vi "Authenticate.vi"(8 "error in (no error)":errorcluster, 10 "Authentication Inputs":T2, 11 "SOL Auth in":refnum<class "SOL Auth.lvclass">) -> (0 "error out":errorcluster, 2 "Authentication Outputs":T1, 3 "SOL Auth out":refnum<class "SOL Auth.lvclass">)   [LabVIEW 2020, in "Summer of LabVIEW.lvlib" / "SOL Auth.lvclass"]
uses:
  SOL Auth.lvclass
  <vilib>/IlluminatedG/IG HTTP Server/HTTP Server/Authentication Inputs.ctl
  <vilib>/IlluminatedG/IG HTTP Server/HTTP Server/Session/Session.lvclass
  <vilib>/IlluminatedG/IG HTTP Utils/HTTP Utils/Request/Request.lvclass
  <vilib>/IlluminatedG/IG HTTP Server/HTTP Server/User Provider/User Provider.lvclass
  <vilib>/IlluminatedG/IG HTTP Server/HTTP Server/Password Encoder/Password Encoder.lvclass
  <vilib>/IlluminatedG/IG HTTP Server/HTTP Server/Authentication Outputs.ctl
  <vilib>/IlluminatedG/IG HTTP Server/HTTP Server/User/User.lvclass
  Data Types/Login JSON.ctl
  Summer of LabVIEW.lvlib
  <vilib>/IlluminatedG/IG HTTP Server/HTTP Server/HTTP Server.lvlib
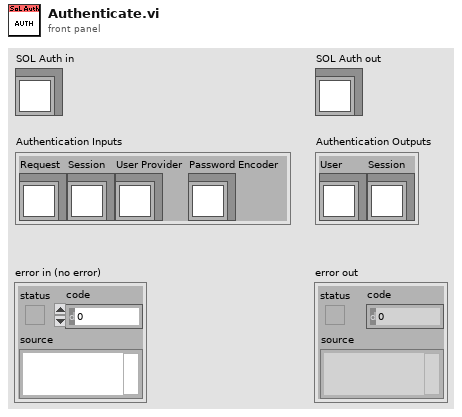
[diagram p1: front panel]
types:
  T1 = typedef "HTTP Server.lvlib/Authentication Outputs.ctl" = cluster{"User":refnum<class "User.lvclass">, "Session":refnum<class "Session.lvclass">}
  T2 = typedef "HTTP Server.lvlib/Authentication Inputs.ctl" = cluster{"Request":refnum<class "Request.lvclass">, "Session":refnum<class "Session.lvclass">, "User Provider":refnum<class "User Provider.lvclass">, "Password Encoder":refnum<class "Password Encoder.lvclass">}
  T3 = typedef "Summer of LabVIEW.lvlib/Login JSON.ctl" = cluster{"Email":string, "Password":string, "CSRF":string}
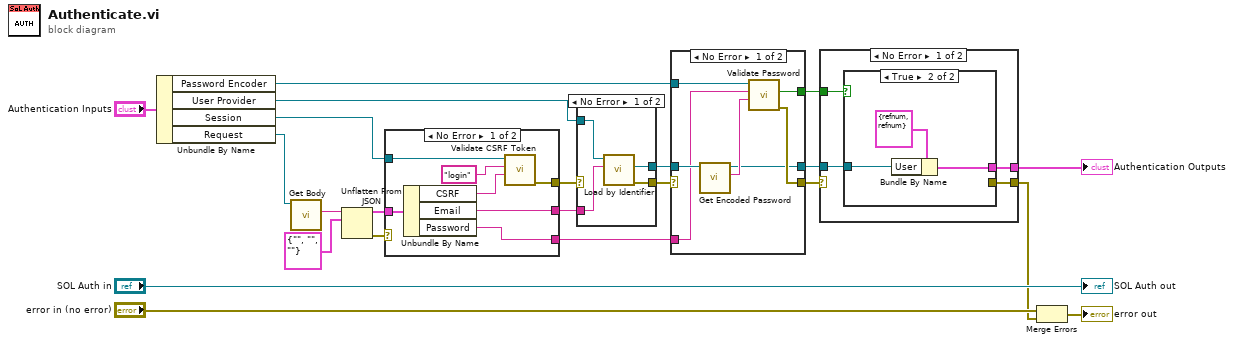
[diagram p0: block diagram]
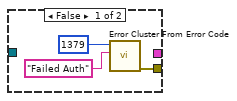
[diagram p2: hidden frame]
diagram:
  n1 = Unbundle By Name("Authentication Inputs") -> ("Password Encoder"=w6:refnum<class "Password Encoder.lvclass">, "User Provider"=w13:refnum<class "User Provider.lvclass">, "Session"=w15:refnum<class "Session.lvclass">, "Request"=w19:refnum<class "Request.lvclass">)
  n2 = call <vilib>:"Get Body.vi"("Request in"=w19) -> ("Body"=w18:string)  [unwired: 8 in, 2 out]
  n3 = Unflatten From JSON(JSON string=w18, type and defaults=T3 {"Email"="", "Password"="", "CSRF"=""} ("Login JSON")) -> (value=w16:T3, error out=w10:errorcluster)  [unwired: 5 in]
  n4 = case shown="No Error" w10 {
    selector: w10 -> [_ w30]
    tunnel: w16 -> [w29 _]
    tunnel: w15 -> [w28 _]
    tunnel: [w25 w30] -> w12
    tunnel: [w24 _] -> w11
    tunnel: [w23 _] -> w7
    frame No Error {
      n5 = Unbundle By Name(w29) -> ("CSRF"=w26:string, "Email"=w24:string, "Password"=w23:string)
      n6 = call <vilib>:"Validate CSRF Token.vi"("Token"=w26, "Token ID"="login", "Session In"=w28) -> ("error out"=w25:errorcluster)  [unwired: 7 in, 1 out]
    }
    frame Error {
    }
  }
  n7 = case shown="No Error" w12 {
    selector: w12 -> [_ w35]
    tunnel: [w32 w35] -> w8
    tunnel: w11 -> [w33 _]
    tunnel: w13 -> [w34 _]
    tunnel: [w31 _] -> w9
    frame No Error {
      n8 = call-dynamic "Load by Identifier.vi"("Identifier"=w33, "User Provider in"=w34) -> ("error out"=w32:errorcluster, "User"=w31:refnum<class "User.lvclass">)  [unwired: 7 in, 1 out]
    }
    frame Error {
    }
  }
  n9 = case shown="No Error" w8 {
    selector: w8 -> [_ w43]
    tunnel: w9 -> [w42 _]
    tunnel: w7 -> [w39 _]
    tunnel: w6 -> [w40 _]
    tunnel: [w38 w43] -> w5
    tunnel: [w37 _] -> w4
    tunnel: [w36 _] -> w3
    frame No Error {
      n10 = call-dynamic "Get Encoded Password.vi"("User in"=w42) -> ("Encoded Password"=w41:string, "User out"=w37:refnum<class "User.lvclass">)  [unwired: 8 in, 1 out]
      n11 = call-dynamic "Validate Password.vi"("Encoded Password"=w41, "Plain Password"=w39, "Password Encoder in"=w40) -> ("error out"=w38:errorcluster, "Valid"=w36:bool)  [unwired: 6 in, 1 out]
    }
    frame Error {
    }
  }
  n12 = case shown="No Error" w5 {
    selector: w5 -> [_ w54]
    tunnel: w4 -> [w46 _]
    tunnel: w3 -> [w47 _]
    tunnel: [w44 w54] -> w2
    tunnel: [w45 _] -> w1
    frame No Error {
      n13 = case shown="True" w47 {
        tunnel: w46 -> [_ w53]
        tunnel: [_ w52] -> w45
        tunnel: [w48 _] -> w44
        frame False {
          n14 = call <vilib>:"Error Cluster From Error Code.vi"("error message (\"\")"="Failed Auth" ("error message (\"\")"), "error code (0)"=1379) -> ("error out"=w48:errorcluster)  [unwired: 7 in]
        }
        frame True {
          n15 = Bundle By Name(cluster=T1 {"User"=refnum, "Session"=refnum} ("Authentication Outputs"), "User"=w53) -> (w52:T1)
        }
      }
    }
    frame Error {
    }
  }
  "Authentication Outputs" <- w1
  n16 = Merge Errors("error in (no error)", w2) -> (→"error out":errorcluster)
  "SOL Auth out" <- "SOL Auth in"
